vi "GetXResolution.vi"() -> (3 "x+y":i32)   [LabVIEW 2016]
uses:
  Robot Global Data.vi
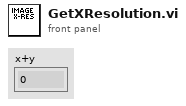
[diagram p1: front panel]
types:
  T1 = typedef "WPI_CameraImageSize.ctl" = enum16{"640x480", "320x240", "160x120", "Custom"}
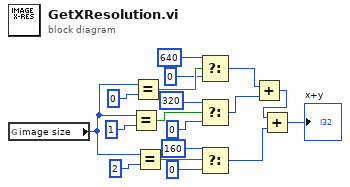
[diagram p0: block diagram]
diagram:
  n1 = global read "Robot Global Data.vi" "image size"() -> (w9:T1)
  n2 = Equal?(x=w9, y=1) -> (x = y?=w13:bool)
  n3 = Equal?(x=w9, y=0) -> (x = y?=w16:bool)
  n4 = Equal?(x=w9, y=2) -> (x = y?=w8:bool)
  n5 = Select(t=640, s=w16, f=0) -> (s? t:f=w5:i32)
  n6 = Select(t=320, s=w13, f=0) -> (s? t:f=w4:i32)
  n7 = Select(t=160, s=w8, f=0) -> (s? t:f=w2:i32)
  n8 = Add(x=w5, y=w4) -> (x+y=w3:i32)
  n9 = Add(x=w3, y=w2) -> (x+y=→"x+y":i32)
